vi "__Alicat SD_Hardware_Module.vi"(5 "Used ?":bool=TRUE, 7 "Command":T2, 8 "error in (no error)":errorcluster, 9 "SetPoint (64000=FullScale)":i32=32000 min=0 max=64000 step=1, 10 "Address":string="A", 11 "VISA resource name":refnum<visa-resource-name>="COM6") -> (0 "error out":errorcluster, 1 "ParsedReading":T1={"ID"="", "Pressure"=13.55, "Temperature"=28.56, "Volumetric"=-1.9, "Mass"=-1.7, "SetPoint"=250.0, "Gas"=""} {"SetPoint" format="%.2f"; "Mass" format="%.2f"; "Volumetric" format="%.2f"; "Temperature" format="%.2f"; "Pressure" format="%.2f"}, 2 "AlicatResponse":string="A +013.53 +023.20 +0000.0 +0000.0 0250.0     Air\r", 3 "Timeout":bool)   [LabVIEW 2017]
uses:
  __Alicat SD_Hardware_Module.ctl
  __Alicat SD_ReadingCluster.ctl
  <vilib>/Instr/_visa.llb/VISA Configure Serial Port (Instr).vi
panel:
  in  "Timeout(s)":dbl=2.0
  # "Input Data"
  # "Output Data"
  # "ESTE NO FUNCIONA. USAR Ver2"
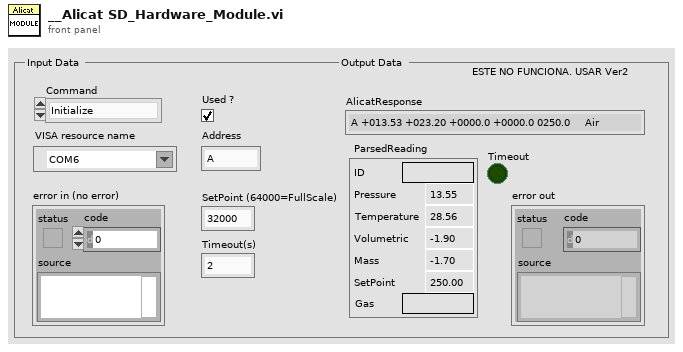
[diagram p1: front panel]
types:
  T1 = typedef "__Alicat SD_ReadingCluster.ctl" = cluster{"ID":string, "Pressure":sgl, "Temperature":sgl, "Volumetric":sgl, "Mass":sgl, "SetPoint":sgl, "Gas":string}
  T2 = typedef "__Alicat SD_Hardware_Module.ctl" = enum16{"Initialize", "Send Setpoint", "Read Data", "Change Address", "Shutdown"}
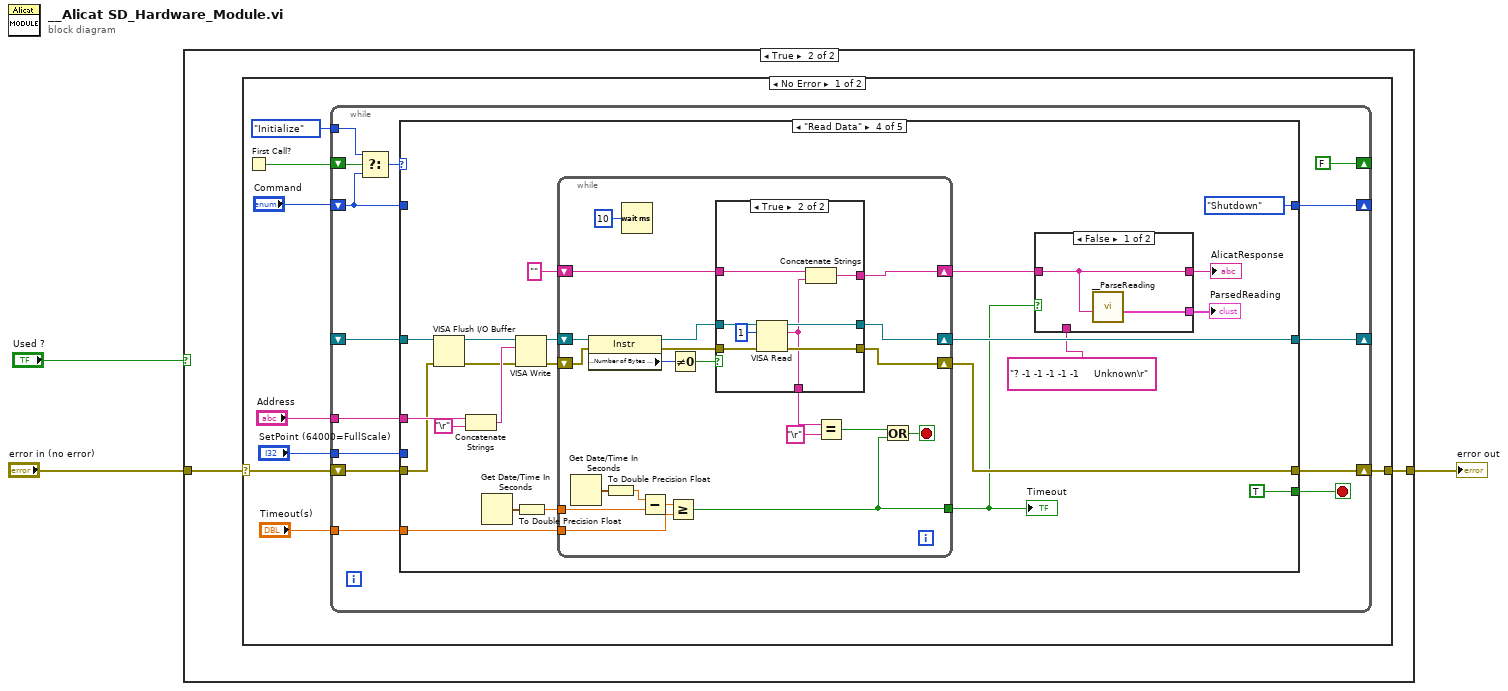
[diagram p0: block diagram]
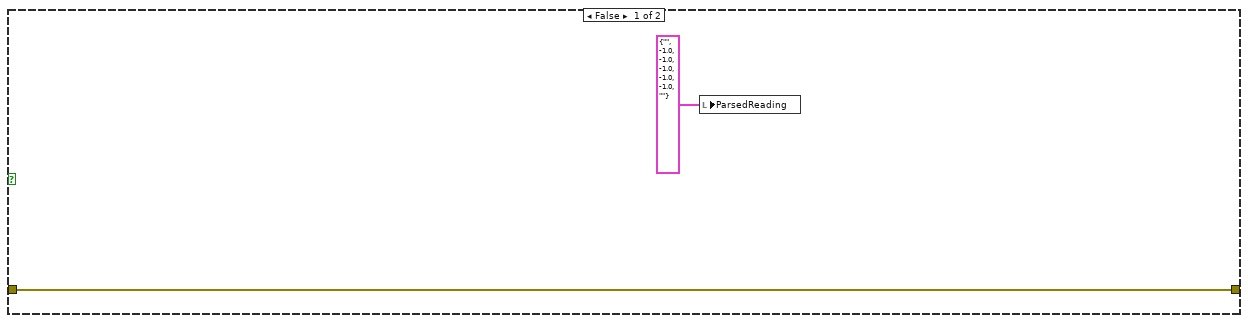
[diagram p2: hidden frame]
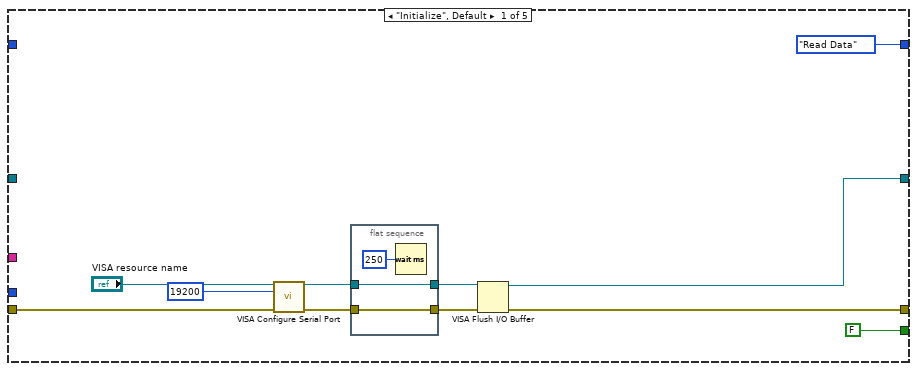
[diagram p3: hidden frame]
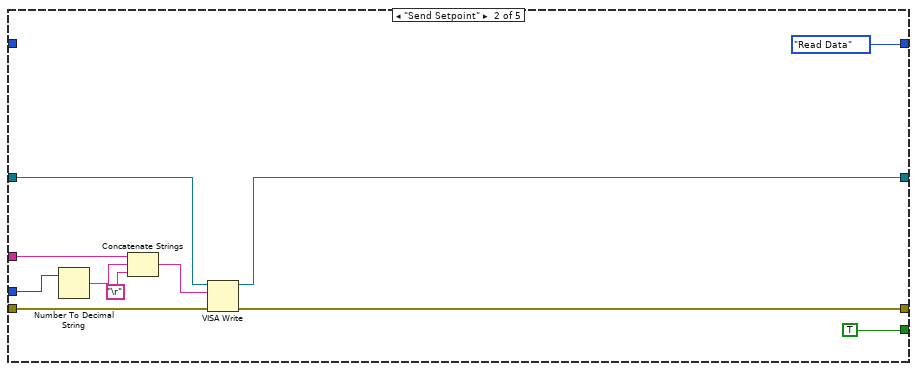
[diagram p4: hidden frame]
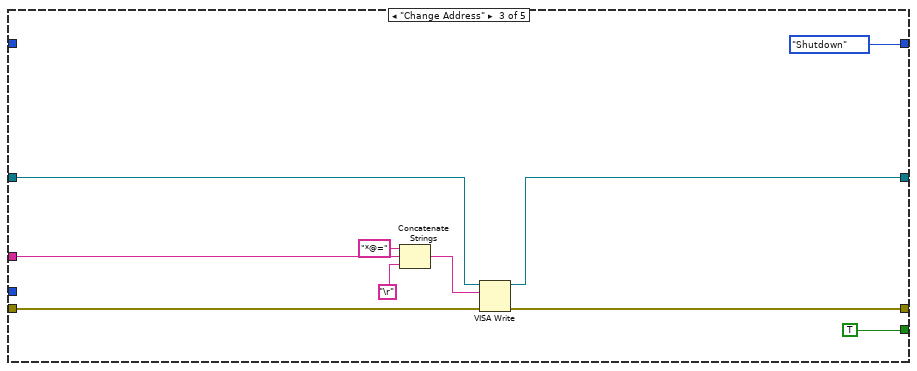
[diagram p5: hidden frame]
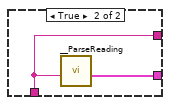
[diagram p6: hidden frame]
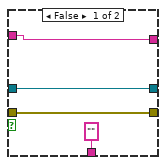
[diagram p7: hidden frame]
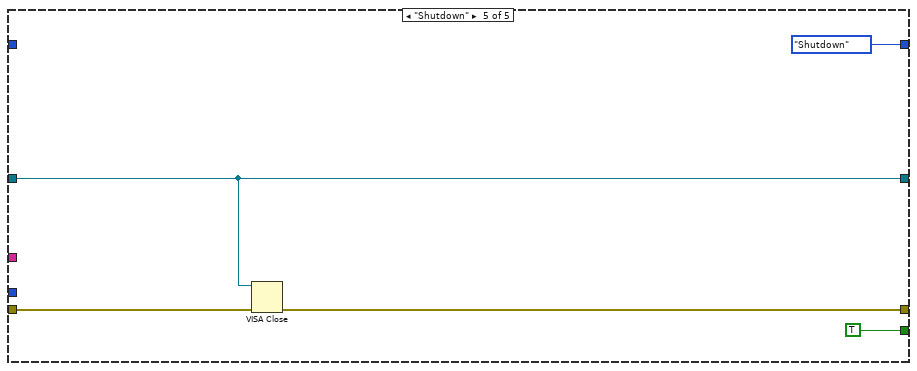
[diagram p8: hidden frame]
diagram:
  n1 = case shown="True" "Used ?" {
    tunnel: "error in (no error)" -> [w5 w7]
    tunnel: [w5 w6] -> w2
    frame False {
      n2 = local write "ParsedReading"(T1 {"ID"="", "Pressure"=-1.0, "Temperature"=-1.0, "Volumetric"=-1.0, "Mass"=-1.0, "SetPoint"=-1.0, "Gas"=""} ("ParsedReading")) -> ()
    }
    frame True {
      n3 = case shown="No Error" w7 {
        selector: w7 -> [w13 w129]
        tunnel: [w12 w129] -> w6
        frame No Error {
          n4 = First Call?() -> (First Call?: T/F=w15:bool)
          n5 = while {
            shift-right: [w21] -> _
            shift-left: "Command" -> [w22]
            shift-right: [w24] -> w12
            shift-left: w13 -> [w25]
            shift-right: [FALSE ("First Call?: T/F")] -> _
            shift-left: w15 -> [w29]
            tunnel: __Alicat_SD_Hardware_Module."Initialize" ("t") -> [w28]
            shift-right: [w19] -> _
            shift-left: _ -> [w20]
            tunnel: "Address" -> [w18]
            tunnel: "SetPoint (64000=FullScale)" -> [w17]
            tunnel: "Timeout(s)" -> [w16]
            stop <- w26 stop-if-true
            n6 = Select(t=w28, s=w29, f=w22) -> (s? t:f=w27:T2)
            n7 = case shown="\"Read Data\"" w27 {
              tunnel: [FALSE TRUE TRUE TRUE TRUE] -> w26
              tunnel: w25 -> [w37 w52 w62 w68 w126]
              tunnel: [w31 w51 w61 w79 w125] -> w24
              tunnel: w22 -> [_ _ _ _ _]
              tunnel: [__Alicat_SD_Hardware_Module."Read Data" ("t") __Alicat_SD_Hardware_Module."Read Data" ("t") __Alicat_SD_Hardware_Module."Shutdown" ("t") __Alicat_SD_Hardware_Module."Shutdown" ("t") __Alicat_SD_Hardware_Module."Shutdown" ("t")] -> w21
              tunnel: w20 -> [_ w47 w58 w66 w124]
              tunnel: [w30 w46 w57 w81 w124] -> w19
              tunnel: w18 -> [_ w50 w60 w74 _]
              tunnel: w17 -> [_ w45 _ _ _]
              tunnel: w16 -> [_ _ _ w82 _]
              frame "Initialize", Default {
                n8 = call-poly "VISA Configure Serial Port"("VISA resource name"="VISA resource name", "baud rate (9600)"=u32 19200, "error in (no error)"=w37) -> ("VISA resource name out"=w33:refnum<visa-resource-name>, "error out"=w32:errorcluster)  [unwired: 11 in]
                n9 = flat-sequence {
                  tunnel: w32 -> [w42]
                  tunnel: [w42] -> w35
                  tunnel: w33 -> [w41]
                  tunnel: [w41] -> w34
                  frame #0 {
                    n10 = Wait (ms)(milliseconds to wait=u32 250) -> ()  [unwired: 1 out]
                  }
                }
                n11 = VISA Flush I/O Buffer(VISA resource name=w34, error in (no error)=w35) -> (VISA resource name out=w30:refnum<visa-resource-name>, error out=w31:errorcluster)  [unwired: 1 in]
              }
              frame "Send Setpoint" {
                n12 = Number To Decimal String(number=w45) -> (decimal integer string=w49:string)  [unwired: 1 in]
                n13 = Concatenate Strings(w50, w49, "\r") -> (w48:string)
                n14 = VISA Write(VISA resource name=w47, write buffer=w48, error in (no error)=w52) -> (VISA resource name out=w46:refnum<visa-resource-name>, error out=w51:errorcluster)  [unwired: 1 out]
              }
              frame "Change Address" {
                n15 = Concatenate Strings("*@=" ("string"), w60, "\r") -> (w59:string)
                n16 = VISA Write(VISA resource name=w58, write buffer=w59, error in (no error)=w62) -> (VISA resource name out=w57:refnum<visa-resource-name>, error out=w61:errorcluster)  [unwired: 1 out]
              }
              frame "Read Data" {
                n17 = VISA Flush I/O Buffer(VISA resource name=w66, error in (no error)=w68) -> (VISA resource name out=w65:refnum<visa-resource-name>, error out=w67:errorcluster)  [unwired: 1 in]
                n18 = Concatenate Strings(w74, "\r") -> (w78:string)
                n19 = Get Date/Time In Seconds() -> (seconds since 1Jan1904=w83:timestamp)
                n20 = VISA Write(VISA resource name=w65, write buffer=w78, error in (no error)=w67) -> (VISA resource name out=w75:refnum<visa-resource-name>, error out=w76:errorcluster)  [unwired: 1 out]
                n21 = To Double Precision Float(number=w83) -> (double precision float=w84:dbl)
                n22 = while {
                  tunnel: w84 -> [w108]
                  shift-right: [w96] -> w81
                  shift-left: w75 -> [w107]
                  shift-right: [w98] -> w79
                  shift-left: w76 -> [w106]
                  tunnel: w82 -> [w104]
                  tunnel: [w102] -> w72
                  shift-right: [w94] -> w73
                  shift-left: "" ("AlicatResponse") -> [w95]
                  stop <- w111 stop-if-true
                  n23 = Get Date/Time In Seconds() -> (seconds since 1Jan1904=w110:timestamp)
                  n24 = property class="Instr"(reference=w107, error in=w106) -> (reference out=w97:refnum<visa-resource-name>, error out=w99:errorcluster, "Serial Settings:Number of Bytes at Serial Port"=w101:u32)
                  n25 = To Double Precision Float(number=w110) -> (double precision float=w109:dbl)
                  n26 = Wait (ms)(milliseconds to wait=u32 10) -> ()  [unwired: 1 out]
                  n27 = Subtract(x=w109, y=w108) -> (x-y=w105:dbl)
                  n28 = Greater Or Equal?(x=w105, y=w104) -> (x >= y?=w102:bool)
                  n29 = Not Equal To 0?(x=w101) -> (x != 0?=w100:bool)
                  n30 = case shown="True" w100 {
                    tunnel: w99 -> [w114 w123]
                    tunnel: [w114 w122] -> w98
                    tunnel: w97 -> [w115 w121]
                    tunnel: [w115 w120] -> w96
                    tunnel: w95 -> [w113 w119]
                    tunnel: [w113 w118] -> w94
                    tunnel: ["" ("read buffer") w117] -> w93
                    frame False {
                    }
                    frame True {
                      n31 = VISA Read(VISA resource name=w121, byte count=u32 1, error in (no error)=w123) -> (VISA resource name out=w120:refnum<visa-resource-name>, read buffer=w117:string, error out=w122:errorcluster)  [unwired: 1 out]
                      n32 = Concatenate Strings(w119, w117) -> (w118:string)
                    }
                  }
                  n33 = Equal?(x=w93, y="\r") -> (x = y?=w91:bool)
                  n34 = Or(x=w91, y=w102) -> (x .or. y?=w111:bool)
                }
                "Timeout" <- w72
                n35 = case shown="False" w72 {
                  tunnel: w73 -> [w88 _]
                  tunnel: [w88 w89] -> w71
                  tunnel: [w87 w90] -> w70
                  tunnel: "? -1 -1 -1 -1 -1     Unknown\r" ("AlicatResponse") -> [_ w89]
                  frame False {
                    n36 = call "__ParseReading.vi"("AlicatResponse"=w88) -> ("ParsedReading"=w87:T1)  [unwired: 9 in, 1 out]
                  }
                  frame True {
                    n37 = call "__ParseReading.vi"("AlicatResponse"=w89) -> ("ParsedReading"=w90:T1)  [unwired: 9 in, 1 out]
                  }
                }
                "AlicatResponse" <- w71
                "ParsedReading" <- w70
              }
              frame "Shutdown" {
                n38 = VISA Close(VISA resource name=w124, error in (no error)=w126) -> (error out=w125:errorcluster)
              }
            }
          }
        }
        frame Error {
        }
      }
    }
  }
  "error out" <- w2
